vi "Autonomous.vi"(8 "error in":errorcluster, 11 "Auto Step":T1[](array[typedef])) -> ()   [LabVIEW 2017]
uses:
  TypeDefAuto.ctl
  TypeDefEnumSelection.ctl
  <vilib>/Rock Robotics/WPI/Solenoid/WPI_SolenoidValue.ctl
  <vilib>/Rock Robotics/WPI/Utilities/WPI_GetSetVariantRefNum.vi
  <vilib>/Rock Robotics/WPI/Solenoid/WPI_SolenoidSetEnum.vi
  <vilib>/Rock Robotics/WPI/RobotDrive/WPI_RobotDriveArcadeDrive_Standard(NoSaturation).vi
panel:
  out "millisecond timer value":u32
  out "millisecond timer value 2":u32
  out "step":i32
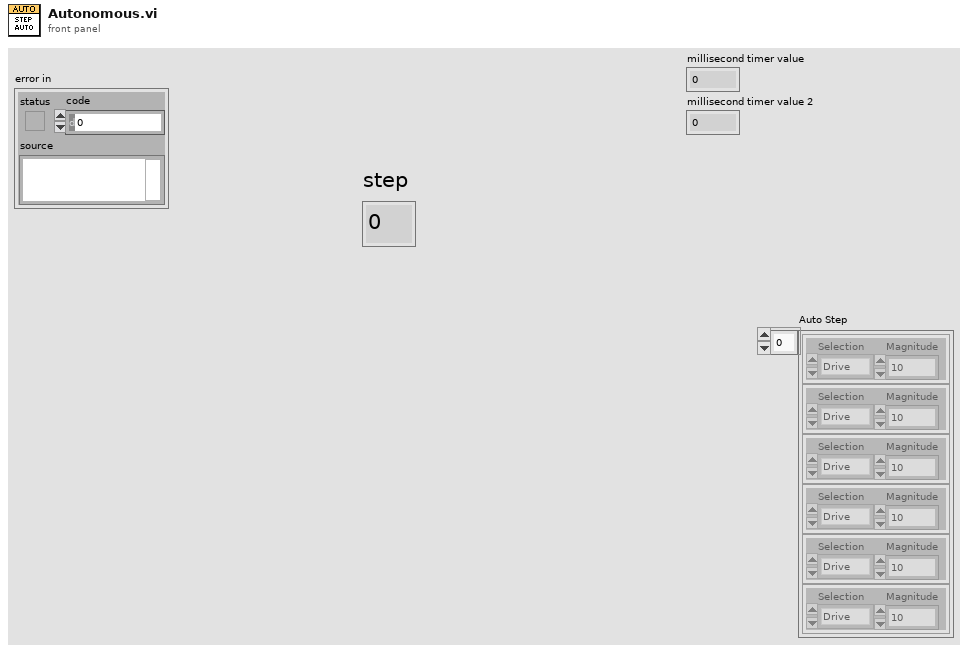
[diagram p1: front panel]
types:
  T1 = typedef "TypeDefAuto.ctl" = cluster{"Selection":T2, "Magnitude":dbl}
  T2 = typedef "TypeDefEnumSelection.ctl" = enum16{"Intake", "Drive", "Turn", "Lift", "Eject", "Wait", "RaiseDrop", "FastDrive", "VisionDrive", "TimedDrive"}
  T3 = typedef "WPI_SolenoidValue.ctl" = enum16{"Off", "On", "Forward", "Reverse"}
  T4 = typedef "WPI_SolenoidDevRef.ctl" = cluster{"DevStatus":errorcluster, "Pneumatics Control Module":u8, "Forward Solenoid Channel":T5, "Reverse Solenoid Channel":T5}
  T5 = typedef "WPI_SolenoidChannel.ctl" = enum8{"Solenoid 0", "Solenoid 1", "Solenoid 2", "Solenoid 3", "Solenoid 4", "Solenoid 5", "Solenoid 6", "Solenoid 7", "Invalid"}
  T6 = typedef "WPI_RobotDriveDevRef.ctl" = cluster{"DevStatus":errorcluster, "Motors[]":T7[], "Square Inputs":bool, "Max Output":dbl}
  T7 = typedef "WPI_MotorControlDeviceRef.ctl" = cluster{"DeviceStatus":errorcluster, "Type":T8, "PWM":cluster{"PWM Channel":T9, "DeadBand":T10}, "CAN":cluster{"Device Number":u8, "SetOutput VI Ref":variant, "GetOutput VI Ref":variant, "Enable VI Ref":variant, "Disable VI Ref":variant, "Data":variant}, "Invert":bool, "DIO PWM":cluster{"PWM \"Enable\" Channel":T9, "DIOChannel":T11, "PWM Rate":dbl}}
  T8 = typedef "WPI_MotorControlType.ctl" = enum16{"PWM", "CAN", "DIO PWM"}
  T9 = typedef "FPGA_DIOPWMChannel.ctl" = enum8{"PWM 0", "PWM 1", "PWM 2", "PWM 3", "PWM 4", "PWM 5", "PWM 6", "PWM 7", "PWM 8", "PWM 9", "PWM MXP 0", "PWM MXP 1", "PWM MXP 2", "PWM MXP 3", "PWM MXP 4", "PWM MXP 5", "PWM MXP 6", "PWM MXP 7", "PWM MXP 8", "PWM MXP 9", "Invalid"}
  T10 = typedef "WPI_PWMDeadband.ctl" = cluster{"Name":string, "maxPositivePwm":i32, "minPositivePwm":i32, "centerPwm":i32, "maxNegativePwm":i32, "minNegativePwm":i32, "angularRange":u16}
  T11 = typedef "FPGA_DIOChannel.ctl" = enum8{"DIO 0", "DIO 1", "DIO 2", "DIO 3", "DIO 4", "DIO 5", "DIO 6", "DIO 7", "DIO 8", "DIO 9", "DIO MXP 0", "DIO MXP 1", "DIO MXP 2", "DIO MXP 3", "DIO MXP 4", "DIO MXP 5", "DIO MXP 6", "DIO MXP 7", "DIO MXP 8", "DIO MXP 9", "DIO MXP 10", "DIO MXP 11", "DIO MXP 12", "DIO MXP 13", "DIO MXP 14", "DIO MXP 15", "SPI Port CS1", "SPI Port CS2", "SPI Port CS3", "SPI Port MISO", "SPI Port MOSI", "Invalid"}
  T12 = typedef "WPI_GyroDevRef.ctl" = cluster{"DevStatus":errorcluster, "Analog Channel":T13, "Gain (VoltsPerDegree/Second)":dbl, "Gyro Type":enum16{"Analog", "XRS450"}, "Handle":i32, "SPI Bus":T14, "Device Found":bool, "Sample Rate":dbl, "Calibrate On Open":bool, "Offset":dbl}
  T13 = typedef "FPGA_AIChannel.ctl" = enum8{"AI 0", "AI 1", "AI 2", "AI 3", "AI MXP 0", "AI MXP 1", "AI MXP 2", "AI MXP 3", "Invalid"}
  T14 = typedef "spi_bus.ctl" = enum16{"SPI On-Board, CS0", "SPI On-Board, CS1", "SPI On-Board, CS2", "SPI On-Board, CS3", "SPI MXP", "Invalid"}
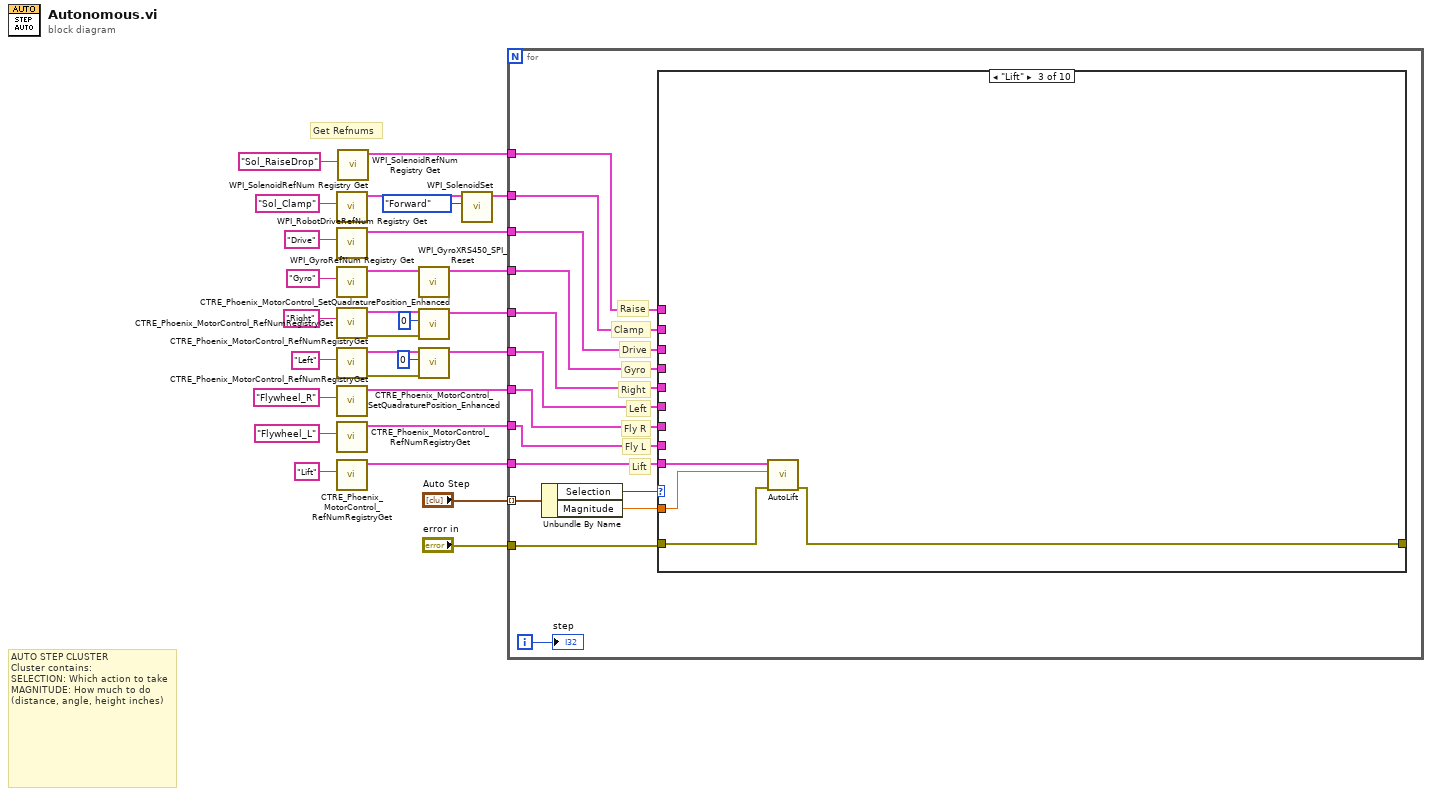
[diagram p0: block diagram]
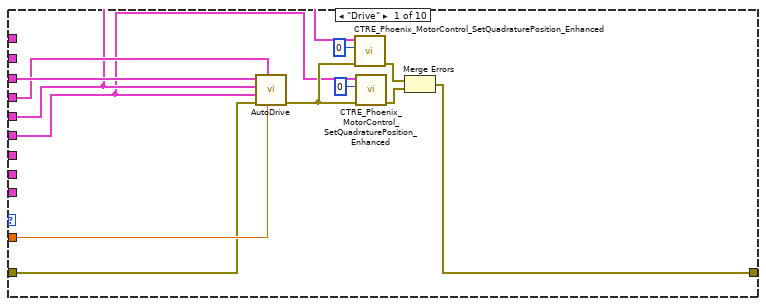
[diagram p2: hidden frame]
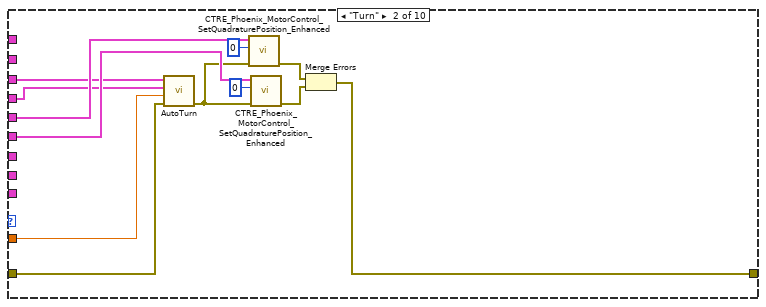
[diagram p3: hidden frame]
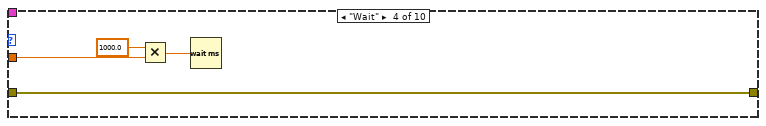
[diagram p4: hidden frame]
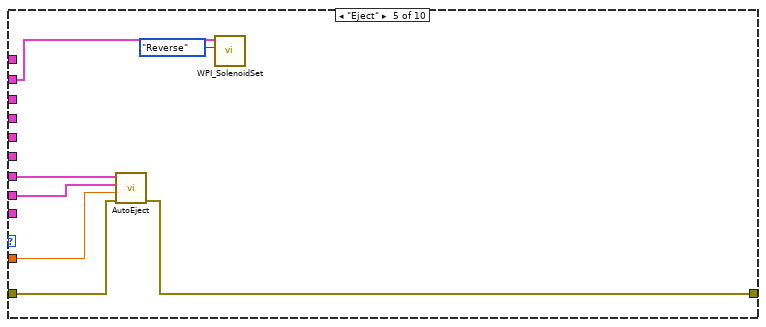
[diagram p5: hidden frame]
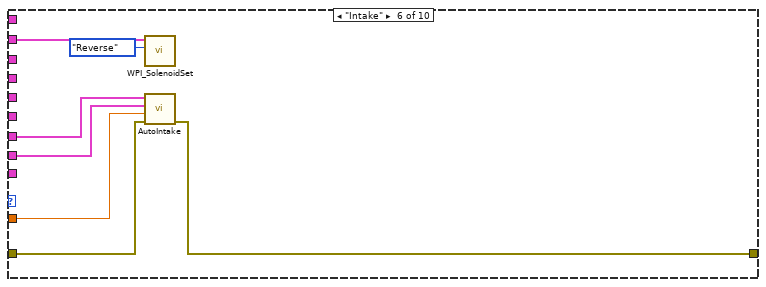
[diagram p6: hidden frame]
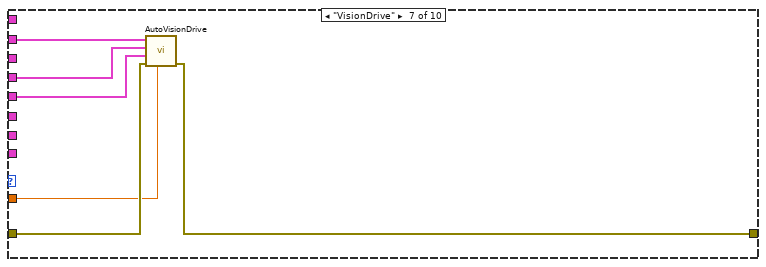
[diagram p7: hidden frame]
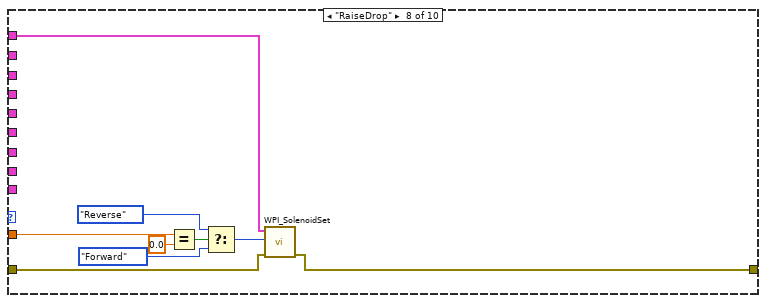
[diagram p8: hidden frame]
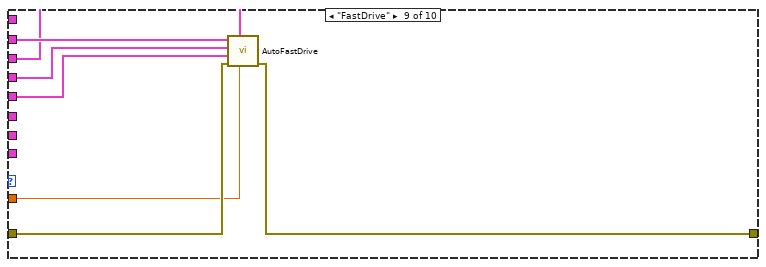
[diagram p9: hidden frame]
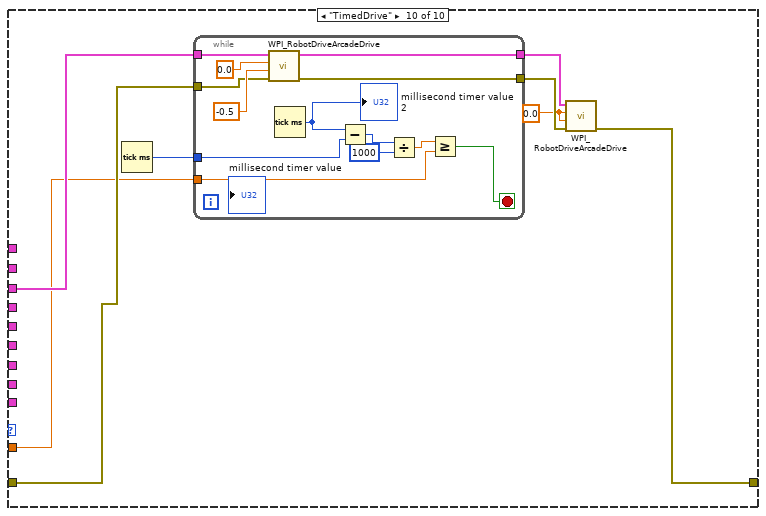
[diagram p10: hidden frame]
diagram:
  # "Get Refnums"
  # "AUTO STEP CLUSTER\nCluster contains:\nSELECTION: Which action to take\nMAGNITUDE: How much to do\n(distance, angle, height inches)"
  n1 = call <vilib>:"WPI_SolenoidRefNum Registry Get.vi"("refnum name"="Sol_Clamp") -> ("SolenoidDevRef"=w3:T4)  [unwired: 9 in, 1 out]
  n2 = call <vilib>:"WPI_RobotDriveRefNum Registry Get.vi"("refnum name"="Drive") -> ("RobotDriveDevRef"=w23:T6)  [unwired: 9 in, 1 out]
  n3 = call <vilib>:"WPI_GyroRefNum Registry Get.vi"("refnum name"="Gyro") -> ("GyroDevRef"=w9:T12)  [unwired: 9 in, 1 out]
  n4 = call <vilib>:"CTRE_Phoenix_MotorControl_RefNumRegistryGet.vi"("refnum name"="Right") -> ("error out"=w7:errorcluster, "PhoenixMotorControlDevRef"=w14:T7)  [unwired: 9 in]
  n5 = call <vilib>:"CTRE_Phoenix_MotorControl_RefNumRegistryGet.vi"("refnum name"="Left") -> ("error out"=w6:errorcluster, "PhoenixMotorControlDevRef"=w12:T7)  [unwired: 9 in]
  n6 = call <vilib>:"CTRE_Phoenix_MotorControl_RefNumRegistryGet.vi"("refnum name"="Flywheel_R") -> ("PhoenixMotorControlDevRef"=w20:T7)  [unwired: 9 in, 1 out]
  n7 = call <vilib>:"CTRE_Phoenix_MotorControl_RefNumRegistryGet.vi"("refnum name"="Flywheel_L") -> ("PhoenixMotorControlDevRef"=w17:T7)  [unwired: 9 in, 1 out]
  n8 = call <vilib>:"CTRE_Phoenix_MotorControl_RefNumRegistryGet.vi"("refnum name"="Lift") -> ("PhoenixMotorControlDevRef"=w19:T7)  [unwired: 9 in, 1 out]
  n9 = call <vilib>:"WPI_SolenoidRefNum Registry Get.vi"("refnum name"="Sol_RaiseDrop") -> ("SolenoidDevRef"=w1:T4)  [unwired: 9 in, 1 out]
  n10 = call <vilib>:"WPI_GyroXRS450_SPI_Reset.vi"("GyroDevRef"=w9) -> ("GyroDevRef"=w8:T12)  [unwired: 9 in, 1 out]
  n11 = call <vilib>:"CTRE_Phoenix_MotorControl_SetQuadraturePosition_Enhanced.vi"("error in (no error)"=w7, "New Position"=0, "PhoenixMotorControlDevRef"=w14) -> ("PhoenixMotorControlDevRef"=w13:T7)  [unwired: 7 in, 1 out]
  n12 = call <vilib>:"CTRE_Phoenix_MotorControl_SetQuadraturePosition_Enhanced.vi"("error in (no error)"=w6, "New Position"=0, "PhoenixMotorControlDevRef"=w12) -> ("PhoenixMotorControlDevRef"=w11:T7)  [unwired: 7 in, 1 out]
  n13 = call-poly <vilib>:"WPI_SolenoidSet.vi"("Value"=WPI_SolenoidValue."Forward", "SolenoidDevRef"=w3) -> ("SolenoidDevRef"=w2:T4)  [unwired: 8 in, 1 out]
  n14 = for {
    tunnel: "Auto Step" -> [w43] mode=indexing
    tunnel: "error in" -> [w40]
    tunnel: w11 -> [w33]
    tunnel: w13 -> [w34]
    tunnel: w8 -> [w32]
    tunnel: w23 -> [w39]
    tunnel: w20 -> [w38]
    tunnel: w19 -> [w37]
    tunnel: w17 -> [w36]
    tunnel: w2 -> [w31]
    tunnel: w1 -> [w30]
    i -> [w35]
    # "Raise"
    # "Lift"
    # "Fly L"
    # "Fly R"
    # "Left"
    # "Right"
    # "Gyro"
    # "Drive"
    # "Clamp"
    n15 = Unbundle By Name(w43) -> ("Selection"=w42:T2, "Magnitude"=w41:dbl)
    n16 = case shown="\"Lift\"" w42 {
      tunnel: w41 -> [w55 w58 w68 w75 w82 w83 w90 w104 w105 w117]
      tunnel: w40 -> [w54 w57 w70 w72 w81 w89 w95 w97 w111 w118]
      tunnel: w33 -> [w47 w64 _ _ _ _ w93 _ w106 _]
      tunnel: w34 -> [w48 w65 _ _ _ _ w92 _ w107 _]
      tunnel: w32 -> [w49 w59 _ _ _ _ _ _ w108 _]
      tunnel: w39 -> [w50 w60 _ _ _ _ w91 _ w109 w119]
      tunnel: w38 -> [_ _ _ _ w80 w85 _ _ _ _]
      tunnel: w37 -> [_ _ w71 _ _ _ _ _ _ _]
      tunnel: w36 -> [_ _ _ _ w79 w84 _ _ _ _]
      tunnel: w31 -> [_ _ _ _ w76 w86 _ _ _ _]
      tunnel: [w44 w61 w69 w72 w78 w88 w94 w98 w110 w112] -> _
      tunnel: w30 -> [_ _ _ _ _ _ _ w96 _ _]
      frame "Drive" {
        n17 = call "AutoDrive.vi"("Distance (Inches)"=w55, "GyroDevRef"=w49, "error in"=w54, "LeftDevRef"=w47, "RightDevRef"=w48, "DriveDevRef"=w50) -> ("error out"=w51:errorcluster)  [unwired: 5 in]
        n18 = call <vilib>:"CTRE_Phoenix_MotorControl_SetQuadraturePosition_Enhanced.vi"("error in (no error)"=w51, "New Position"=0, "PhoenixMotorControlDevRef"=w48) -> ("error out"=w45:errorcluster)  [unwired: 7 in, 1 out]
        n19 = call <vilib>:"CTRE_Phoenix_MotorControl_SetQuadraturePosition_Enhanced.vi"("error in (no error)"=w51, "New Position"=0, "PhoenixMotorControlDevRef"=w47) -> ("error out"=w46:errorcluster)  [unwired: 7 in, 1 out]
        n20 = Merge Errors(w45, w46) -> (w44:errorcluster)
      }
      frame "Turn" {
        n21 = call "AutoTurn.vi"("error in (no error)"=w57, "Setpoint"=w58, "GyroDevRef"=w59, "RobotDriveDevRef"=w60) -> ("error out"=w56:errorcluster)  [unwired: 7 in]
        n22 = call <vilib>:"CTRE_Phoenix_MotorControl_SetQuadraturePosition_Enhanced.vi"("error in (no error)"=w56, "New Position"=0, "PhoenixMotorControlDevRef"=w65) -> ("error out"=w62:errorcluster)  [unwired: 7 in, 1 out]
        n23 = call <vilib>:"CTRE_Phoenix_MotorControl_SetQuadraturePosition_Enhanced.vi"("error in (no error)"=w56, "New Position"=0, "PhoenixMotorControlDevRef"=w64) -> ("error out"=w63:errorcluster)  [unwired: 7 in, 1 out]
        n24 = Merge Errors(w62, w63) -> (w61:errorcluster)
      }
      frame "Lift" {
        n25 = call "AutoLift.vi"("error in (no error)"=w70, "Setpoint"=w68, "Lift DevRef"=w71) -> ("error out"=w69:errorcluster)  [unwired: 8 in]
      }
      frame "Wait" {
        n26 = Multiply(x=1000.0, y=w75) -> (x*y=w74:dbl)
        n27 = Wait (ms)(milliseconds to wait=w74) -> ()  [unwired: 1 out]
      }
      frame "Eject" {
        n28 = call "AutoEject.vi"("error in (no error)"=w81, "Time"=w82, "Left Flywheel DevRef"=w79, "Right Flywheel DevRef"=w80) -> ("error out"=w78:errorcluster)  [unwired: 7 in]
        n29 = call-poly <vilib>:"WPI_SolenoidSet.vi"("Value"=WPI_SolenoidValue."Reverse", "SolenoidDevRef"=w76) -> ()  [unwired: 8 in, 2 out]
      }
      frame "Intake" {
        n30 = call-poly <vilib>:"WPI_SolenoidSet.vi"("Value"=WPI_SolenoidValue."Reverse", "SolenoidDevRef"=w86) -> ()  [unwired: 8 in, 2 out]
        n31 = call "AutoIntake.vi"("error in (no error)"=w89, "Speed"=w83, "Left Flywheel DevRef"=w84, "Right Flywheel DevRef"=w85) -> ("error out"=w88:errorcluster)  [unwired: 7 in]
      }
      frame "VisionDrive" {
        n32 = call "AutoVisionDrive.vi"("Distance (Inches)"=w90, "error in"=w95, "LeftDevRef"=w93, "RightDevRef"=w92, "DriveDevRef"=w91) -> ("error out"=w94:errorcluster)  [unwired: 6 in]
      }
      frame "RaiseDrop" {
        n33 = Equal?(x=w104, y=0.0) -> (x = y?=w102:bool)
        n34 = Select(t=WPI_SolenoidValue."Reverse" ("Value"), s=w102, f=WPI_SolenoidValue."Forward" ("Value")) -> (s? t:f=w100:T3)
        n35 = call-poly <vilib>:"WPI_SolenoidSet.vi"("error in (no error)"=w97, "Value"=w100, "SolenoidDevRef"=w96) -> ("error out"=w98:errorcluster)  [unwired: 7 in, 1 out]
      }
      frame "FastDrive" {
        n36 = call "AutoFastDrive.vi"("Distance (Inches)"=w105, "GyroDevRef"=w108, "error in"=w111, "LeftDevRef"=w106, "RightDevRef"=w107, "DriveDevRef"=w109) -> ("error out"=w110:errorcluster)  [unwired: 5 in]
      }
      frame "TimedDrive" {
        w114 = 0.0 ("Y axis value")
        n37 = Tick Count (ms)() -> (millisecond timer value=w113:u32)
        n38 = while {
          tunnel: w119 -> [w129]
          tunnel: w118 -> [w128]
          tunnel: w117 -> [w124]
          tunnel: [w122] -> w116
          tunnel: [w121] -> w115
          tunnel: w113 -> [w120]
          stop <- w123 stop-if-true
          n39 = call-poly <vilib>:"WPI_RobotDriveArcadeDrive.vi"("error in (no error)"=w128, "Y axis value"=-0.5, "X axis value"=0.0, "RobotDriveDevRef"=w129) -> ("error out"=w121:errorcluster, "RobotDriveDevRef"=w122:T6)  [unwired: 5 in, 1 out]
          n40 = Tick Count (ms)() -> (millisecond timer value=w132:u32)
          "millisecond timer value 2" <- w132
          n41 = Subtract(x=w132, y=w120) -> (x-y=w127:u32)
          n42 = Divide(x=w127, y=u32 1000) -> (x/y=w125:dbl)
          n43 = Greater Or Equal?(x=w125, y=w124) -> (x >= y?=w123:bool)
        }
        n44 = call-poly <vilib>:"WPI_RobotDriveArcadeDrive.vi"("error in (no error)"=w115, "Y axis value"=w114, "X axis value"=w114, "RobotDriveDevRef"=w116) -> ("error out"=w112:errorcluster)  [unwired: 5 in, 2 out]
      }
    }
    "step" <- w35
  }
